vi "Get FPGA Properties.vi"(6 "FPGA Target":T1, 8 "error in (no error)":errorcluster, 11 "Item Ref in":T2 format="%.0x") -> (0 "error out":errorcluster, 1 "TargetClass":string, 2 "Bitfile Path":path, 3 "Item Ref out":T2 format="%.0x")   [LabVIEW 2016, in "Scan Engine Custom Device.lvlib"]
uses:
  Scan Engine Custom Device.lvlib
  <vilib>/NI Veristand/Custom Device API/Custom Device Item Ref.ctl
  Type Defs/FPGA Target.ctl
  Globals/Property Strings.vi
  <vilib>/NI Veristand/Custom Device API/Get Item Property (Path).vi
  <vilib>/NI Veristand/Custom Device API/Get Item Property (String).vi
  <vilib>/NI Veristand/Custom Device API/Custom Device API.lvlib
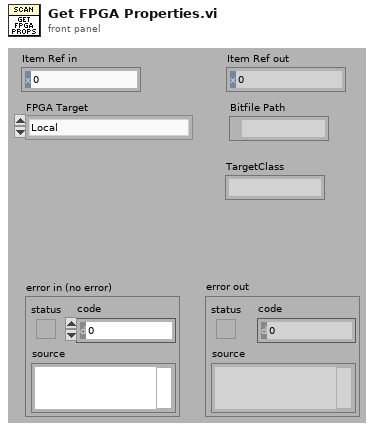
[diagram p1: front panel]
types:
  T1 = typedef "Scan Engine Custom Device.lvlib/FPGA Target.ctl" = enum16{"Local", "EtherCAT"}
  T2 = typedef "Custom Device API.lvlib/Custom Device Item Ref.ctl" = u64
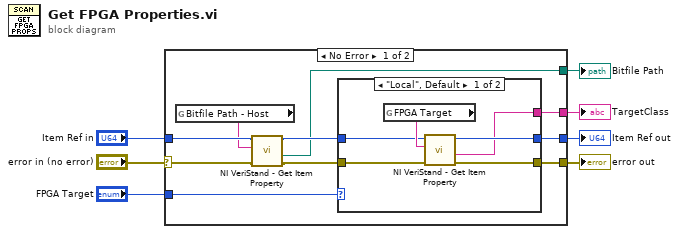
[diagram p0: block diagram]
diagram:
  n1 = case shown="No Error" "error in (no error)" {
    selector: "error in (no error)" -> [w12 w27]
    tunnel: [w15 w27] -> w6
    tunnel: [w16 w26] -> w5
    tunnel: "Item Ref in" -> [w14 w26]
    tunnel: "FPGA Target" -> [w17 _]
    tunnel: [w9 _] -> w2
    tunnel: [w8 _] -> w1
    frame No Error {
      n2 = global read "Property Strings.vi" "Bitfile Path - Host"() -> (w10:string)
      n3 = call-poly <vilib>:"NI VeriStand - Get Item Property.vi"("error in (no error)"=w12, "Property Name"=w10, "Item Ref in"=w14) -> ("error out"=w11:errorcluster, "Value"=w8:path, "Item Ref out"=w13:T2)  [unwired: 5 in, 1 out]
      n4 = case shown="\"Local\", Default" w17 {
        tunnel: w13 -> [w22 w25]
        tunnel: w11 -> [w21 w24]
        tunnel: [w19 w25] -> w16
        tunnel: [w20 w24] -> w15
        tunnel: [w18 _] -> w9
        frame "Local", Default {
          n5 = global read "Property Strings.vi" "FPGA Target"() -> (w23:string)
          n6 = call-poly <vilib>:"NI VeriStand - Get Item Property.vi"("error in (no error)"=w21, "Property Name"=w23, "Item Ref in"=w22) -> ("error out"=w20:errorcluster, "Value"=w18:string, "Item Ref out"=w19:T2)  [unwired: 5 in, 1 out]
        }
        frame "EtherCAT" {
        }
      }
    }
    frame Error {
    }
  }
  "Item Ref out" <- w5
  "error out" <- w6
  "TargetClass" <- w2
  "Bitfile Path" <- w1
